vi "pmacGetRes.vi"(9 "字符串":string, 10 "PCOMMSERVERLib.IPmacDevice":refnum<k7>, 11 "Digital输入":refnum<vi>) -> (3 "pAnswer":string)   [LabVIEW 2018]
panel:
  out "错误输出":errorcluster
  out "引用输出":refnum<vi>
  in  "错误输入（无错误）":errorcluster
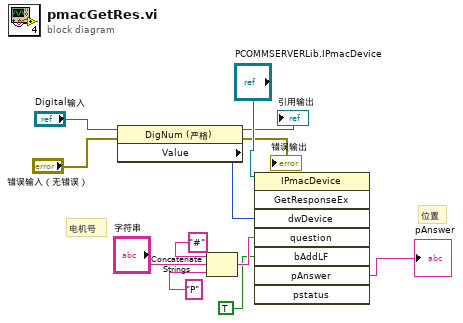
[diagram p0: block diagram]
diagram:
  # "位置"
  # "电机号"
  n1 = property class="DigNum (严格)"(reference="Digital输入", error in="错误输入（无错误）") -> (reference out=→"引用输出":refnum<vi>, error out=→"错误输出":errorcluster, "Value"=w9:i32)
  n2 = Concatenate Strings("#", "字符串", "P") -> (w6:string)
  n3 = invoke class="IPmacDevice" method="GetResponseEx"(reference="PCOMMSERVERLib.IPmacDevice", "dwDevice"=w9, "question"=w6, "bAddLF"=TRUE) -> ("pAnswer"=→"pAnswer":string)  [unwired: 4 in, 7 out]
